vi "串口初始化.vi"(0 "VISA resource name":refnum<visa-resource-name>="COM1", 1 "flow control":u16(ring) items=["None"=0, "XON/XOFF"=1, "RTS/CTS"=2, "DTR/DSR"=4], 2 "XON Character":u8=17 format="%.0x", 3 "termination char\n(0xA = '\\n' = LF)":u8=10 format="%.0x", 5 "baud rate":u32=9600, 7 "data bits":u16=8 min=5 max=8 step=1, 9 "parity":u16(ring) items=["None", "Odd", "Even", "Mark", "Space"], 11 "stop bits":u16(ring)=10 items=["1.0"=10, "1.5"=15, "2.0"=20], 12 "Input buffer size":u32=4096 caption="Input\nbuffer size", 13 "XOFF Character":u8=19 format="%.0x", 14 "timeout (ms)":u32=10000) -> (4 "VISA resource name out":refnum<visa-resource-name>, 6 "错误输出":errorcluster)   [LabVIEW 2017]
uses:
  <vilib>/Instr/_visa.llb/VISA Configure Serial Port (Instr).vi
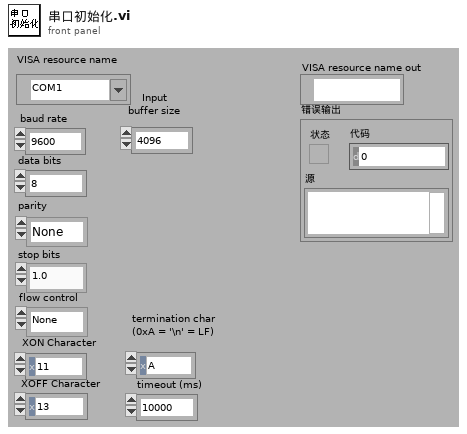
[diagram p1: front panel]
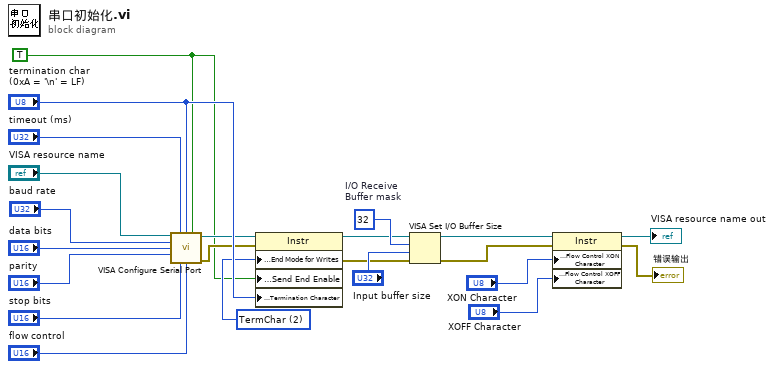
[diagram p0: block diagram]
diagram:
  w4 = TRUE ("End read on termination character?")
  w5 = u16 2 items=["None", "LastBit", "TermChar", "Break"] ("Serial Settings:Serial End Mode for Writes")
  w17 = u16 32  # I/O Receive Buffer mask
  n1 = call-poly "VISA Configure Serial Port"("VISA resource name"="VISA resource name", "timeout (10sec)"="timeout (ms)", "termination char\n(0xA = '\\n' = LF)"="termination char\n(0xA = '\\n' = LF)", "Enable Termination\nChar (T)"=w4, "baud rate (9600)"="baud rate", "data bits (8)"="data bits", "parity (0:none)"="parity", "stop bits (10: 1 bit)"="stop bits", "flow control (0:none)"="flow control") -> ("VISA resource name out"=w6:refnum<visa-resource-name>, "error out"=w8:errorcluster)  [unwired: 5 in]
  n2 = property class="Instr"(reference=w6, error in=w8, "Serial Settings:End Mode for Writes"=w5, "Message Based Settings:Send End Enable"=w4, "Message Based Settings:Termination Character"="termination char\n(0xA = '\\n' = LF)") -> (reference out=w1:refnum<visa-resource-name>, error out=w7:errorcluster)
  n3 = VISA Set I/O Buffer Size(VISA resource name=w1, mask (16)=w17, size (4096)="Input buffer size", error in (no error)=w7) -> (VISA resource name out=w13:refnum<visa-resource-name>, error out=w12:errorcluster)
  n4 = property class="Instr"(reference=w13, error in=w12, "Serial Settings:Flow Control XON Character"="XON Character", "Serial Settings:Flow Control XOFF Character"="XOFF Character") -> (reference out=→"VISA resource name out":refnum<visa-resource-name>, error out=→"错误输出":errorcluster)
